vi "Enumerate Chassis.vi"(8 "error in (no error)":errorcluster) -> (0 "error out":errorcluster, 3 "Devices (ordered)":tag[](array[tag]))   [LabVIEW 2019, in "Instrument.DAQ.lvclass"]
uses:
  Instrument.DAQ.lvclass
  <vilib>/nisyscfg/Close (Hardware).vi
  <vilib>/nisyscfg/Close (System).vi
  <vilib>/nisyscfg/nisyscfg.lvlib
  <resource>/objmgr/nicontrollersysapi.rc
  <resource>/objmgr/nisysapi.rc
  <resource>/objmgr/daqmx.rc
panel:
  out "PxiChassis Numbers":u32[](array[numeric])
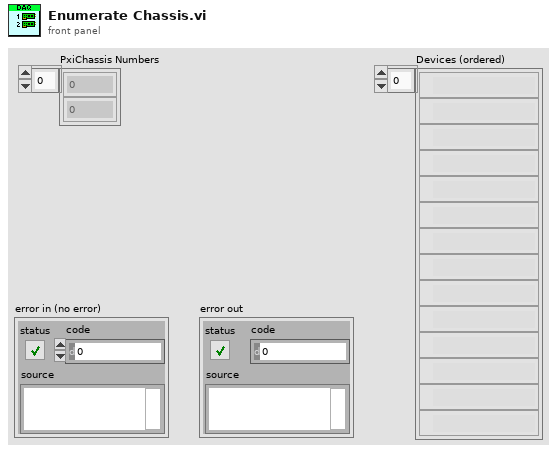
[diagram p1: front panel]
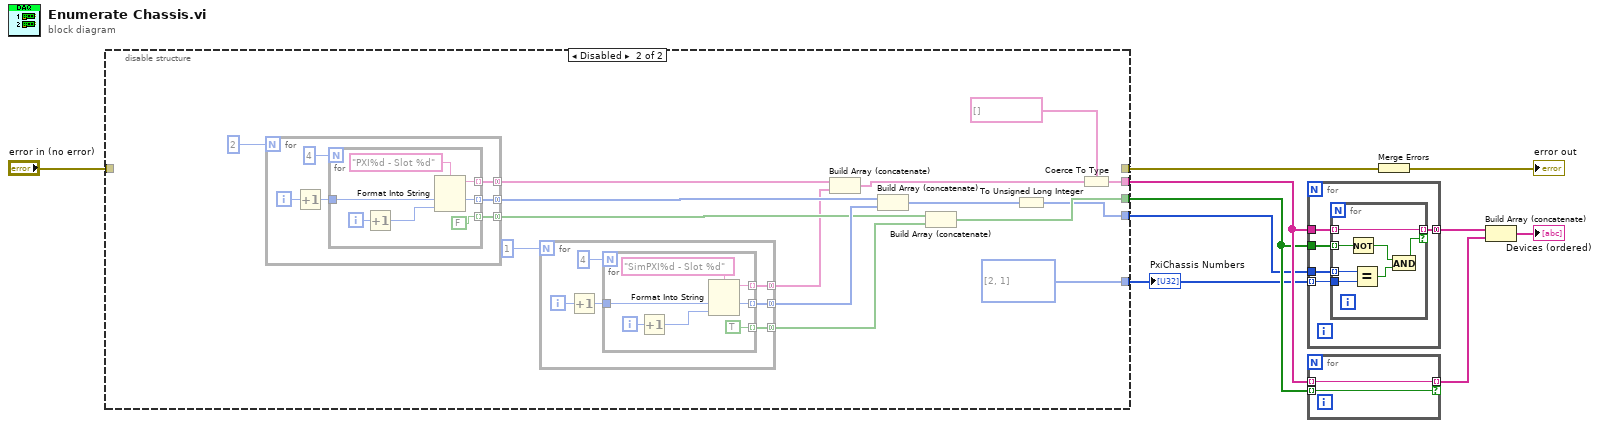
[diagram p0: block diagram]
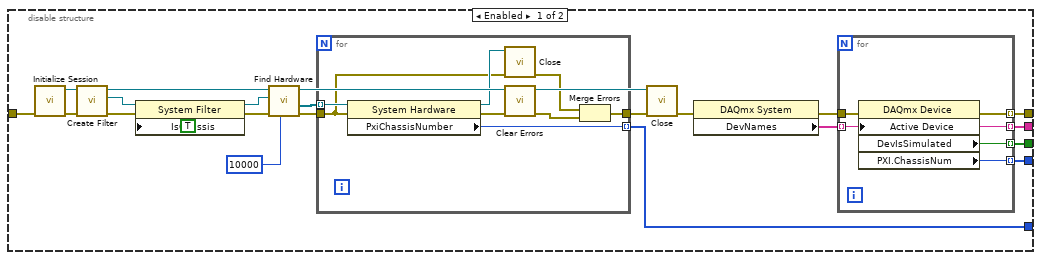
[diagram p2: hidden frame]
diagram:
  n1 = disable-structure shown="Disabled" {
    disable-tunnel: "error in (no error)" -> [w32 _]
    disable-tunnel: [w31 _] -> w8
    disable-tunnel: [w30 u32[] [2, 1] ("PxiChassis Numbers")] -> w1
    disable-tunnel: [w28 w59] -> w5
    disable-tunnel: [w12 w47] -> w3
    disable-tunnel: [w11 w46] -> w2
    frame Enabled {
      n2 = call <vilib>:"Initialize Session.vi"("error in (no error)"=w32) -> ("error out"=w22:errorcluster, "Session out"=w20:refnum<k21>)  [unwired: 9 in]
      n3 = call <vilib>:"Create Filter.vi"("error in (no error)"=w22, "Session in"=w20) -> ("error out"=w18:errorcluster, "Filter out"=w19:refnum<k20>, "Session out"=w21:refnum<k21>)  [unwired: 7 in]
      n4 = property class="System Filter"(reference=w19, error in=w18, "IsChassis"=TRUE ("Is Chassis")) -> (reference out=w24:refnum<k20>, error out=w25:errorcluster)
      n5 = call <vilib>:"Find Hardware.vi"("Remote Timeout (300,000 ms)"=u32 10000, "error in (no error)"=w25, "Filter in"=w24, "Session in"=w21) -> ("error out"=w16:errorcluster, "Resources out"=w15:refnum<k20>[], "Session out"=w13:refnum<k21>)  [unwired: 4 in, 1 out]
      n6 = for {
        tunnel: w15 -> [w45] mode=indexing
        tunnel: w16 -> [w38]
        tunnel: [w43] -> w17
        tunnel: [w39] -> w30 mode=indexing
        n7 = property class="System Hardware"(reference=w45, error in=w38) -> (reference out=w44:refnum<k20>, error out=w42:errorcluster, "PxiChassisNumber"=w39:u32)
        n8 = call-poly <vilib>:"Close.vi"("error in (no error)"=w38, "Resource in"=w44) -> ("error out"=w40:errorcluster)  [unwired: 9 in]
        n9 = call <vilib>:"Clear Errors.vi"("error in (no error)"=w42) -> ("error out"=w41:errorcluster)  [unwired: 5 in, 1 out]
        n10 = Merge Errors(w40, w41) -> (w43:errorcluster)
      }
      n11 = call-poly <vilib>:"Close.vi"("error in (no error)"=w17, "Session in"=w13) -> ("error out"=w29:errorcluster)  [unwired: 9 in]
      n12 = property class="DAQmx System"(error in=w29) -> (error out=w27:errorcluster, "DevNames"=w26:tag[])  [unwired: 1 in, 1 out]
      n13 = for {
        tunnel: w26 -> [w35] mode=indexing
        tunnel: w27 -> [w37]
        tunnel: [w34] -> w31 mode=indexing
        tunnel: [w35] -> w28 mode=indexing
        tunnel: [w36] -> w12 mode=indexing
        tunnel: [w33] -> w11 mode=indexing
        n14 = property class="DAQmx Device"(error in=w37, "Active Device"=w35) -> (error out=w34:errorcluster, "DevIsSimulated"=w36:bool, "PXI.ChassisNum"=w33:u32)  [unwired: 1 in, 1 out]
      }
    }
    frame Disabled {
      n15 = for {
        N: 2 -> [_]
        tunnel: [w78] -> w53 mode=concatenating
        tunnel: [w76] -> w52 mode=concatenating
        tunnel: [w73] -> w51 mode=concatenating
        i -> [w75]
        n16 = Increment(x=w75) -> (x+1=w74:i32)
        n17 = for {
          N: 4 -> [_]
          tunnel: [w83] -> w78 mode=indexing
          tunnel: w74 -> [w81]
          tunnel: [w81] -> w76 mode=indexing
          tunnel: [FALSE] -> w73 mode=indexing
          i -> [w84]
          n18 = Increment(x=w84) -> (x+1=w80:i32)
          n19 = Format Into String(format string="PXI%d - Slot %d", w81, w80) -> (resulting string=w83:string)  [unwired: 2 in, 1 out]
        }
      }
      n20 = for {
        N: 1 -> [_]
        tunnel: [w61] -> w50 mode=concatenating
        tunnel: [w65] -> w55 mode=concatenating
        tunnel: [w62] -> w54 mode=concatenating
        i -> [w64]
        n21 = Increment(x=w64) -> (x+1=w63:i32)
        n22 = for {
          N: 4 -> [_]
          tunnel: [w71] -> w61 mode=indexing
          tunnel: w63 -> [w69]
          tunnel: [w69] -> w65 mode=indexing
          tunnel: [TRUE] -> w62 mode=indexing
          i -> [w72]
          n23 = Increment(x=w72) -> (x+1=w68:i32)
          n24 = Format Into String(format string="SimPXI%d - Slot %d", w69, w68) -> (resulting string=w71:string)  [unwired: 2 in, 1 out]
        }
      }
      n25 = Build Array (concatenate)(w53, w50) -> (w48:string[])
      n26 = Build Array (concatenate)(w52, w55) -> (w49:i32[])
      n27 = Build Array (concatenate)(w51, w54) -> (w47:bool[])
      n28 = To Unsigned Long Integer(number=w49) -> (unsigned 32bit integer=w46:u32[])
      n29 = Coerce To Type(0:w48, 1:tag[] []) -> (2:w59:tag[])
    }
  }
  "PxiChassis Numbers" <- w1
  n30 = for {
    tunnel: w5 -> [w89]
    tunnel: w2 -> [w88]
    tunnel: [w87] -> w7 mode=concatenating
    tunnel: w1 -> [w86] mode=indexing
    tunnel: w3 -> [w85]
    n31 = for {
      tunnel: [w96] -> w87 mode=indexing if=w92
      tunnel: w89 -> [w96] mode=indexing
      tunnel: w88 -> [w95] mode=indexing
      tunnel: w86 -> [w94]
      tunnel: w85 -> [w93] mode=indexing
      n32 = Not(x=w93) -> (.not. x?=w91:bool)
      n33 = Equal?(x=w95, y=w94) -> (x = y?=w90:bool)
      n34 = And(x=w91, y=w90) -> (x .and. y?=w92:bool)
    }
  }
  n35 = for {
    tunnel: [w98] -> w4 mode=indexing if=w97
    tunnel: w5 -> [w98] mode=indexing
    tunnel: w3 -> [w97] mode=indexing
  }
  n36 = Merge Errors(w8) -> (→"error out":errorcluster)
  n37 = Build Array (concatenate)(w7, w4) -> (→"Devices (ordered)":tag[])
